vi "Configure Channel.vi"(7 "Enable Channel (True)":bool=TRUE, 8 "error in (no error)":errorcluster, 10 "Cluster":T1={"Channel (0: Channel 1)"=0, "Vertical Coupling (1: DC)"=1, "Probe Attenuation (10: 10X)"=10, "Vertical Range (10.0 V/div)"=10.0, "Vertical Offset (0.0 divs)"=0.0, "Bandwidth (0: MAX Bandwidth)"=0} {"Bandwidth (0: MAX Bandwidth)" items=["MAX Bandwidth", "Unlimited"]; "Probe Attenuation (10: 10X)" items=["1"=1, "10"=10, "20"=20, "50"=50, "100"=100, "500"=500, "1000"=1000]; "Vertical Coupling (1: DC)" items=["AC", "DC", "Ground"]; "Channel (0: Channel 1)" items=["Channel 1", "Channel 2", "Channel 3", "Channel 4", "Math", "Reference A", "Reference B", "Reference C", "Reference D"]}, 11 "Osciloscopio in":refnum<class "Osciloscopio.lvclass">) -> (0 "error out":errorcluster, 3 "Osciloscopio out":refnum<class "Osciloscopio.lvclass">)   [LabVIEW 2020, in "Oscilloscope.lvlib" / "Osciloscopio.lvclass"]
uses:
  Osciloscopio.lvclass
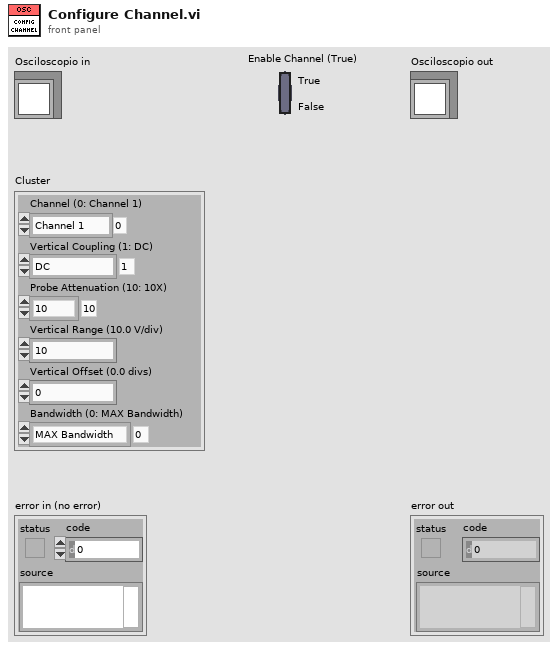
[diagram p1: front panel]
types:
  T1 = cluster{"Channel (0: Channel 1)":i32, "Vertical Coupling (1: DC)":i32, "Probe Attenuation (10: 10X)":i32, "Vertical Range (10.0 V/div)":dbl, "Vertical Offset (0.0 divs)":dbl, "Bandwidth (0: MAX Bandwidth)":i32}
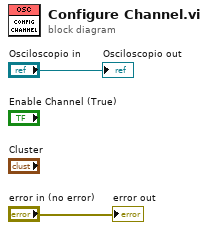
[diagram p0: block diagram]
diagram:
  "error out" <- "error in (no error)"
  "Osciloscopio out" <- "Osciloscopio in"
